vi "IMAQdx_Flea3_set_attrib_coerce.vi"(4 "error in":errorcluster, 5 "value":variant, 6 "attribute":string, 7 "IMAQdx in":T1) -> (0 "error out":errorcluster, 1 "coerced?":bool, 2 "attrib out":variant, 3 "IMAQdx out":T1)   [LabVIEW 2012]
uses:
  <vilib>/userdefined/High Color/IMAQdx.ctl
  <resource>/objmgr/imaqdx.rc
panel:
  out "MaxDBL":dbl format="%#_6e"
  out "MinDBL":dbl format="%#_6e"
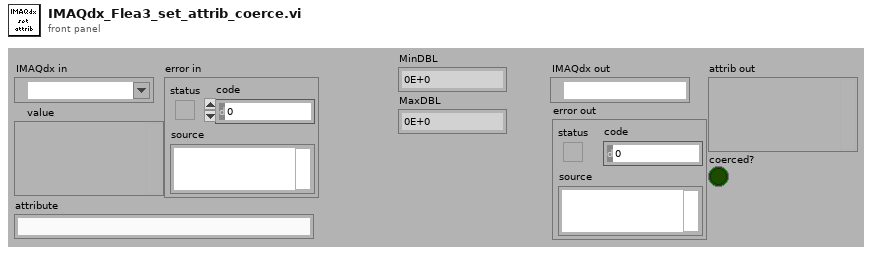
[diagram p1: front panel]
types:
  T1 = typedef "IMAQdx.ctl" = refnum<k21>
  T2 = typedef "Type Descriptor Enumeration__ogtk.ctl" = enum8{"<Null>", "I8", "I16", "I32", "I64", "U8", "U16", "U32", "U64", "SGL", "DBL", "EXT", "CSG", "CDB", "CXT", "0x0F", "0x10", "0x11", "0x12", "0x13", "0x14", "Enum U8", "Enum U16", "Enum U32", "Enum U64", "SGL PQ", "DBL PQ", "EXT PQ", "CSG PQ", "CDB PQ", "CXT PQ", "0x1F", "0x20", "Boolean", "0x22", "0x23", "0x24", "0x25", "0x26", "0x27", "0x28", "0x29", "0x2A", "0x2B", "0x2C", "0x2D", "0x2E", "0x2F", "String", "0x31", "Path", "Pict", "0x34", "0x35", "0x36", "DAQ", "0x38", "0x39", "0x3A", "0x3B", "0x3C", "0x3D", "0x3E", "0x3F", "Array", "0x41", "0x42", "0x43", "0x44", "0x45", "0x46", "0x47", "0x48", "0x49", "0x4A", "0x4B", "0x4C", "0x4D", "0x4E", "0x4F", "Cluster", "0x51", "0x52", "Variant", "Waveform", "0x55", "0x56", "0x57", "0x58", "0x59", "0x5A", "0x5B", "0x5C", "0x5D", "0x5E", "0x5F", "0x60", "0x61", "0x62", "0x63", "0x64", "0x65", "0x66", "0x67", "0x68", "0x69", "0x6A", "0x6B", "0x6C", "0x6D", "0x6E", "0x6F", "Refnum"}
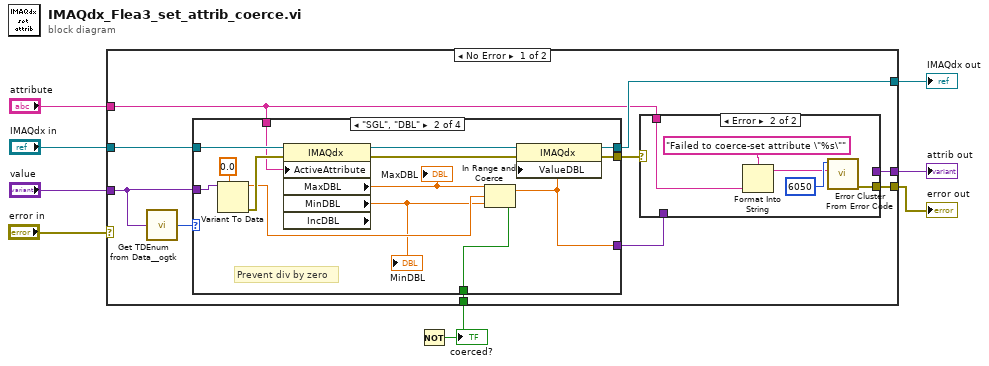
[diagram p0: block diagram]
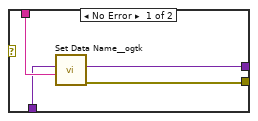
[diagram p2: hidden frame]
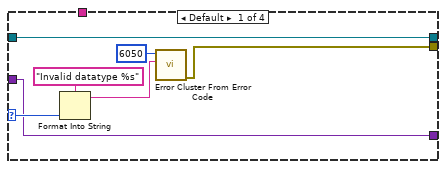
[diagram p3: hidden frame]
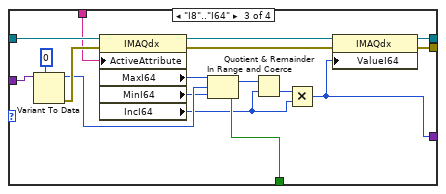
[diagram p4: hidden frame]
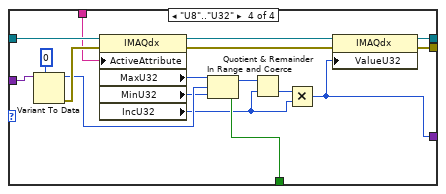
[diagram p5: hidden frame]
diagram:
  n1 = case shown="No Error" "error in" {
    selector: "error in" -> [_ w85]
    tunnel: [w19 w84] -> w9
    tunnel: "IMAQdx in" -> [w18 w84]
    tunnel: "value" -> [w11 _]
    tunnel: "attribute" -> [w15 _]
    tunnel: [w14 w85] -> w5
    tunnel: [w13 _] -> w3
    tunnel: [w12 _] -> w2
    frame No Error {
      n2 = call <userlib>:"Get TDEnum from Data__ogtk.vi"("Data"=w11) -> ("Type Descriptor Enumeration"=w17:T2)  [unwired: 4 in]
      n3 = case shown="\"SGL\", \"DBL\"" w17 {
        selector: w17 -> [w34 _ _ _]
        tunnel: [w35 w39 w56 w73] -> w19
        tunnel: w18 -> [w35 w49 w66 w83]
        tunnel: w11 -> [w29 w47 w64 w81]
        tunnel: w15 -> [_ w45 w62 w79]
        tunnel: [w31 w38 w55 w72] -> w16
        tunnel: [_ w37 w54 w71] -> w12
        tunnel: [w29 w36 w53 w70] -> w10
        frame Default {
          n4 = Format Into String(format string="Invalid datatype %s", w34) -> (resulting string=w30:string)  [unwired: 2 in, 1 out]
          n5 = call <vilib>:"Error Cluster From Error Code.vi"("error message (\"\")"=w30, "error code (0)"=6050) -> ("error out"=w31:errorcluster)  [unwired: 7 in]
        }
        frame "SGL", "DBL" {
          # "Prevent div by zero"
          n6 = Variant To Data(type=0.0 ("ValueU32"), Variant=w47) -> (data=w44:dbl, error out=w46:errorcluster)  [unwired: 1 in]
          n7 = property class="IMAQdx" props=["ActiveAttribute", "MaxDBL", "MinDBL", "IncDBL"](reference=w49, error in=w46, "ActiveAttribute"=w45) -> (reference out=w40:T1, error out=w41:errorcluster, "MaxDBL"=w43:dbl, "MinDBL"=w42:dbl)  [unwired: 1 out]
          "MinDBL" <- w42
          "MaxDBL" <- w43
          n8 = In Range and Coerce(upper limit=w43, x=w44, lower limit=w42) -> (coerced(x)=w36:dbl, In Range?=w37:bool)
          n9 = property class="IMAQdx"(reference=w40, error in=w41, "ValueDBL"=w36) -> (reference out=w39:T1, error out=w38:errorcluster)
        }
        frame "I8".."I64" {
          n10 = Variant To Data(type=i64 0 ("ValueU32"), Variant=w64) -> (data=w61:i64, error out=w63:errorcluster)  [unwired: 1 in]
          n11 = property class="IMAQdx"(reference=w66, error in=w63, "ActiveAttribute"=w62) -> (reference out=w57:T1, error out=w58:errorcluster, "MaxI64"=w60:i64, "MinI64"=w59:i64, "IncI64"=w51:i64)
          n12 = In Range and Coerce(upper limit=w60, x=w61, lower limit=w59) -> (coerced(x)=w52:i64, In Range?=w54:bool)
          n13 = Quotient & Remainder(x=w52, y=w51) -> (floor(x/y)=w50:i64)  [unwired: 1 out]
          n14 = Multiply(x=w50, y=w51) -> (x*y=w53:i64)
          n15 = property class="IMAQdx"(reference=w57, error in=w58, "ValueI64"=w53) -> (reference out=w56:T1, error out=w55:errorcluster)
        }
        frame "U8".."U32" {
          n16 = Variant To Data(type=u32 0 ("ValueU32"), Variant=w81) -> (data=w78:u32, error out=w80:errorcluster)  [unwired: 1 in]
          n17 = property class="IMAQdx"(reference=w83, error in=w80, "ActiveAttribute"=w79) -> (reference out=w74:T1, error out=w75:errorcluster, "MaxU32"=w77:u32, "MinU32"=w76:u32, "IncU32"=w68:u32)
          n18 = In Range and Coerce(upper limit=w77, x=w78, lower limit=w76) -> (coerced(x)=w69:u32, In Range?=w71:bool)
          n19 = Quotient & Remainder(x=w69, y=w68) -> (floor(x/y)=w67:u32)  [unwired: 1 out]
          n20 = Multiply(x=w67, y=w68) -> (x*y=w70:u32)
          n21 = property class="IMAQdx"(reference=w74, error in=w75, "ValueU32"=w70) -> (reference out=w73:T1, error out=w72:errorcluster)
        }
      }
      n22 = case shown="Error" w16 {
        tunnel: w15 -> [w23 w25]
        tunnel: [w22 w24] -> w14
        tunnel: w10 -> [w20 _]
        tunnel: [w21 _] -> w13
        frame No Error {
          n23 = call <userlib>:"Set Data Name__ogtk.vi"("Data Name"=w23, "Data"=w20) -> ("error out"=w22:errorcluster, "Renamed Data"=w21:variant)  [unwired: 8 in]
        }
        frame Error {
          n24 = Format Into String(format string="Failed to coerce-set attribute \"%s\"", w25) -> (resulting string=w26:string)  [unwired: 2 in, 1 out]
          n25 = call <vilib>:"Error Cluster From Error Code.vi"("error message (\"\")"=w26, "error code (0)"=6050) -> ("error out"=w24:errorcluster)  [unwired: 7 in]
        }
      }
    }
    frame Error {
    }
  }
  "IMAQdx out" <- w9
  "error out" <- w5
  "attrib out" <- w3
  n26 = Not(x=w2) -> (.not. x?=→"coerced?":bool)
